vi "Launcher.vi"() -> ()   [LabVIEW 2018]
uses:
  <vilib>/ActorFramework/Message Enqueuer/Message Enqueuer.lvclass
  Counter/Counter/Counter.lvclass
  C:/Program Files (x86)/National Instruments/LabVIEW 2018/vi.lib/ActorFramework/Actor/Actor.lvclass
  Counter/Counter Messages/Increment Msg/Increment Msg.lvclass/Increment Msg.ctl
  <vilib>/ActorFramework/Message Enqueuer/Message Enqueuer.lvclass/Message Enqueuer.ctl
  Counter/Counter Messages/Decrement Msg/Decrement Msg.lvclass/Decrement Msg.ctl
  <vilib>/ActorFramework/Message Enqueuer/Enqueue.vi
  Counter/Counter Messages/Increment Msg/Increment Msg.lvclass
  C:/Program Files (x86)/National Instruments/LabVIEW 2018/vi.lib/ActorFramework/Message/Message.lvclass
  Counter/Counter Messages/Decrement Msg/Decrement Msg.lvclass
  Counter/Counter Messages/Reset Msg/Reset Msg.lvclass
  <vilib>/ActorFramework/Stop Msg/Stop Msg.lvclass
  <vilib>/ActorFramework/Message Priority Queue/Priority Enqueue.vi
  <vilib>/ActorFramework/Actor/Actor.lvclass
panel:
  in  "Select Counter":u32(ring) items=["Select counter", "1"]
  in  "Reset":bool
  in  "Decrement":bool
  in  "Increment":bool
  in  "Launch new counter":bool
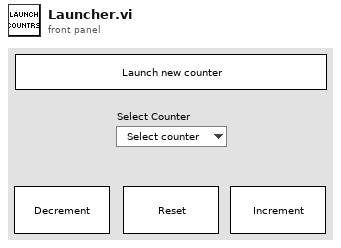
[diagram p1: front panel]
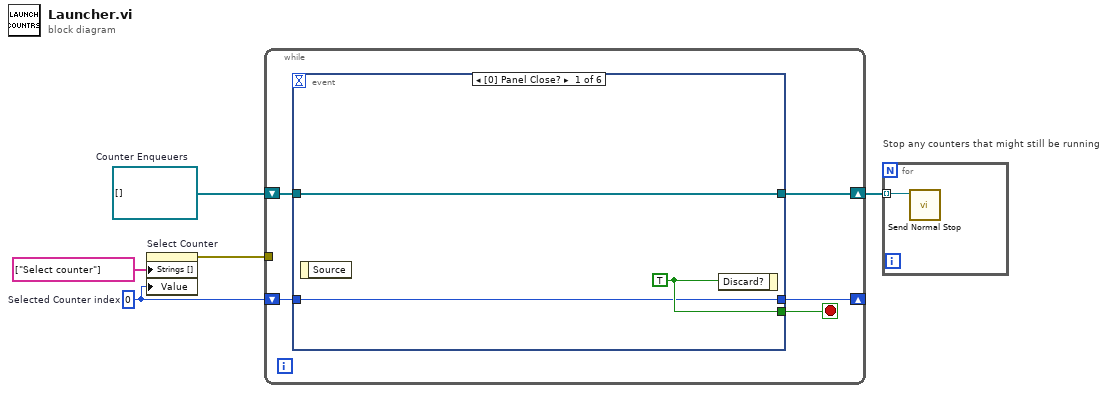
[diagram p0: block diagram]
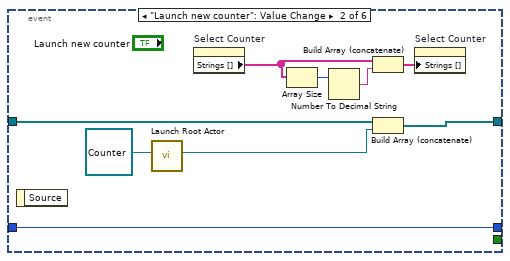
[diagram p2: hidden frame]
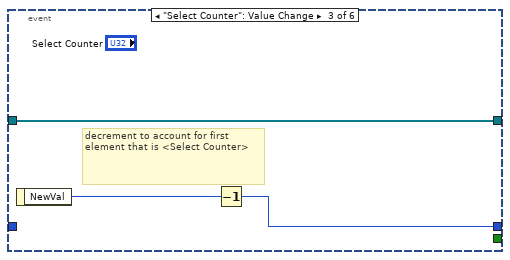
[diagram p3: hidden frame]
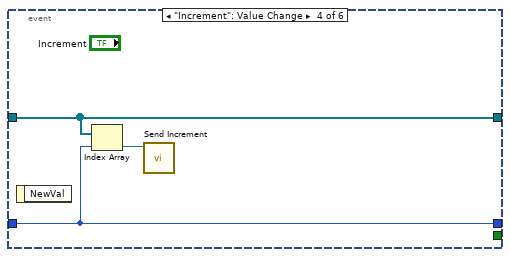
[diagram p4: hidden frame]
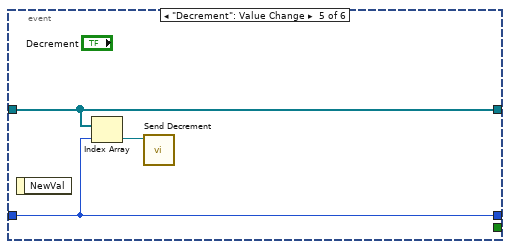
[diagram p5: hidden frame]
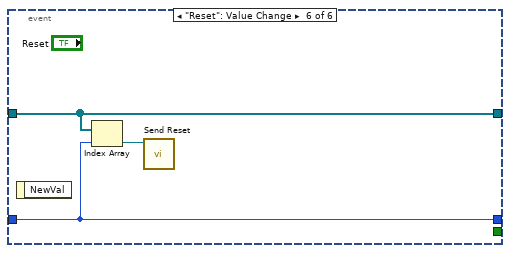
[diagram p6: hidden frame]
diagram:
  w1 = u32 0  # Selected Counter index
  w5 = refnum<class "Message Enqueuer.lvclass">[] []  # Counter Enqueuers
  n1 = property on="Select Counter" class="Ring (strict)"("Strings []"=string[] ["Select counter"], "Value"=w1) -> (error out=w3:errorcluster)  [unwired: 2 in, 1 out]
  n2 = while {
    shift-right: [w9] -> w4
    shift-left: w5 -> [w8]
    shift-right: [w7] -> _
    shift-left: w1 -> [w6]
    tunnel: w3 -> [_]
    stop <- w10 stop-if-true
    n3 = event shown="[0] Panel Close?" {
      selector: _ -> [_ _ _ _ _ _]
      dyn-events: _ -> [_ _ _ _ _ _]
      timeout: _ -> [_ _ _ _ _ _]
      tunnel: [w13 _ _ _ _ _] -> w10
      tunnel: [w12 w19 w25 w28 w31 w34] -> w9
      tunnel: w8 -> [w12 w21 w25 w28 w31 w34]
      tunnel: [w11 w18 w23 w26 w29 w32] -> w7
      tunnel: w6 -> [w11 w18 _ w26 w29 w32]
      event Panel Close? {
        w13 = TRUE ("Discard?")
        n4 = event-data() -> ()  [unwired: 1 in, 1 out]
        n5 = event-data("Discard?"=w13) -> ()  [unwired: 1 in, 1 out]
      }
      event "Launch new counter": Value Change {
        n6 = event-data() -> ()  [unwired: 1 in, 1 out]
        n7 = call <vilib>:"Launch Root Actor.vi"("Actor"=refnum<class "Counter.lvclass"> refnum ("Counter.lvlib:Counter")) -> ("Actor's Enqueuer"=w20:refnum<class "Message Enqueuer.lvclass">)  [unwired: 9 in, 1 out]
        n8 = property on="Select Counter" class="Ring (strict)"() -> ("Strings []"=w17:string[])  [unwired: 2 in, 2 out]
        n9 = Array Size(array=w17) -> (size(s)=w14:i32)
        n10 = Number To Decimal String(number=w14) -> (decimal integer string=w16:string)  [unwired: 1 in]
        n11 = Build Array (concatenate)(w17, w16) -> (w15:string[])
        n12 = Build Array (concatenate)(w21, w20) -> (w19:refnum<class "Message Enqueuer.lvclass">[])
        n13 = property on="Select Counter" class="Ring (strict)"("Strings []"=w15) -> ()  [unwired: 2 in, 2 out]
      }
      event "Select Counter": Value Change {
        # "decrement to account for first element that is <Select Counter>"
        n14 = event-data() -> ("NewVal"=w24:u32)  [unwired: 1 in]
        n15 = Decrement(x=w24) -> (x-1=w23:u32)
      }
      event "Increment": Value Change {
        n16 = event-data() -> ()  [unwired: 1 in, 1 out]
        n17 = Index Array(array=w28, index=w26) -> (element=w27:refnum<class "Message Enqueuer.lvclass">)
        n18 = call "Send Increment.vi"("Message Enqueuer"=w27) -> ()  [unwired: 9 in, 2 out]
      }
      event "Decrement": Value Change {
        n19 = event-data() -> ()  [unwired: 1 in, 1 out]
        n20 = Index Array(array=w31, index=w29) -> (element=w30:refnum<class "Message Enqueuer.lvclass">)
        n21 = call "Send Decrement.vi"("Message Enqueuer"=w30) -> ()  [unwired: 9 in, 2 out]
      }
      event "Reset": Value Change {
        n22 = event-data() -> ()  [unwired: 1 in, 1 out]
        n23 = Index Array(array=w34, index=w32) -> (element=w33:refnum<class "Message Enqueuer.lvclass">)
        n24 = call "Send Reset.vi"("Message Enqueuer"=w33) -> ()  [unwired: 9 in, 2 out]
      }
    }
  }
  n25 = for "Stop any counters that might still be running" {
    tunnel: w4 -> [w35] mode=indexing
    n26 = call <vilib>:"Send Normal Stop.vi"("Message Enqueuer"=w35) -> ()  [unwired: 10 in, 1 out]
  }
